vi "UHR-Fleezers Control (host) - 16.2.2v2.vi"() -> ()   [LabVIEW 2014]
uses:
  <vilib>/rvi/interface/nirviMethod/nirviMethod.xnode
  <vilib>/rvi/interface/nirviCloseFPGA/nirviCloseFPGA.xnode
  <vilib>/express/express analysis/Spectral/XNode/ExpressSpectralMeasurementsBlockNode.xnode
  <vilib>/rvi/interface/nirviReadWriteControl/nirviReadWriteControl.xnode
  <vilib>/Analysis/NI_AALBase.lvlib
  <vilib>/express/express analysis/Spectral/Block/exnSpectralBlock spectral measurements PSD poly.vi
  <vilib>/rvi/interface/nirviOpenFPGA/nirviOpenFPGA.xnode
  <vilib>/Platform/TimedLoop/XDataNode/XDataNode.xnode
  <vilib>/Platform/TimedLoop/XDataNode/nitl_modes.ctl
  <vilib>/Platform/TimedLoop/XDataNode/XDNodeRunTimeDep.lvlib
  <vilib>/Platform/TimedLoop/XDataNode/wakeup.ctl
  <vilib>/Platform/TimedLoop/XDataNode/timing_clust.ctl
  <vilib>/Utility/miscctls.llb/LVPoint32TypeDef.ctl
  <vilib>/userdefined/High Color/nirio_resource_hc.ctl
  openfpgaref.8.6.ctl
  <vilib>/Utility/miscctls.llb/LVMinMaxIncTypeDef.ctl
  <vilib>/vision/NI_Vision_Development_Module.lvlib
  <vilib>/Instr/_visa.llb/VISA Configure Serial Port (Instr).vi
  <vilib>/rvi/errors/niLvFpgaMergeErrorWithErrorCode.vi
  <vilib>/Analysis/baseanly.llb/Mean (DBL).vi
  Duncan Nall/Fluorescence simulation/Global for fluorescence simulation mean (30 samples), (power series).vi
  <vilib>/addons/database/NI_Database_API.lvlib
  <vilib>/vision/Avi.llb/IMAQ AVI2 Refnum.ctl
  <vilib>/gmath/NI_Gmath.lvlib
  <vilib>/addons/database/Connection.llb/DB Tools Open Connec (Path).vi
  <vilib>/sound2/lvsound2.llb/Sound Output Write (DBL Single).vi
  <vilib>/Waveform/WDTOps.llb/WDT Append Waveforms DBL.vi
  <vilib>/express/express analysis/Spectral/Block/exnSpectralBlock spectral measurements PSD WFM.vi
  <vilib>/Waveform/WDTOps.llb/WDT Index Channel DBL.vi
  <vilib>/rvi/errors/niLvFpgaAdjustHostInterfaceError.vi
  <vilib>/FPGAPlugInAG/PCIe-7852R/niLvFpga_ConfigureFifo_PCIe-7852R.vi
  <vilib>/FPGAPlugInAG/PCIe-7852R/niLvFpga_ReadFifo_PCIe-7852R.vi
  <vilib>/FPGAPlugInAG/PCIe-7852R/niLvFpga_Open_PCIe-7852R.vi
  openfpgaref.initrf.ctl
  FPGA Bitfiles/UHR-FleezersInst_FPGATarget_intitializeRFsyn_v1.lvbitx
  <vilib>/FPGAPlugInAG/PCIe-7852R/niLvFpga_Close_PCIe-7852R.vi
  FPGA Bitfiles/UHR-FleezersInst_FPGATarget_UHR-Fleezers_main_16.2.1v3.lvbitx
  <vilib>/FPGAPlugInAG/PCIe-7852R/niLvFpga_Reset_PCIe-7852R.vi
  <vilib>/FPGAPlugInAG/PCIe-7852R/niLvFpga_Run_PCIe-7852R.vi
  NiFpgaLv.dll
  <vilib>/Utility/error.llb/Error Cluster From Error Code.vi
  FPGA Bitfiles/UHR-FleezersInst_FPGATarget_UHR-FleezersCont_RmCmolmxQJQ.lvbitx
  UHR-Fleezers Control (fpga) - avogadro 3.vi
  <vilib>/FPGAPlugInAG/PCIe-7852R/niLvFpga_StopFifo_PCIe-7852R.vi
  <vilib>/FPGAPlugInAG/PCIe-7852R/niLvFpga_StartFifo_PCIe-7852R.vi
  <vilib>/addons/database/Connection.llb/Conn ObjectReference.ctl
  <vilib>/sound2/lvsound2.llb/Sampling Mode.ctl
  <vilib>/sound2/lvsound2.llb/Sound Data Format.ctl
panel:
  out "Read offset current":string(combo)
  out "PSD Y Sum":dbl[](array[numeric])
  out "log file ref":refnum<file>
  out "AL Running":bool
  in  "AL Delay (s)":u32
  in  "Stop assembly line":bool
  in  "Cy5 Fl.  Thresh. (kHz)":dbl=24.5
  in  "Cy3 Fl.  Thresh. (kHz)":dbl=19.0
  in  "Get Fluorophore":bool
  in  "X or Y?":bool=TRUE
  out "Red Fluorophore":bool
  out "Green Fluorophore":bool
  in  "Numeric":dbl
  in  "stop":bool
  in  "Start assembly line":bool
  out "Sigma/Mean 3":dbl=nan caption="Sigma/Mean" format="%#_2g"
  out "Rate sigma (Hz) 3":dbl caption="Sigma (Hz)" format="%0.2f"
  out "APD 3 Rate (Hz)":dbl format="%#_3p"
  out "HP3 Flush Time (s)":dbl=90.0
  out "HP1 Flush Time (s)":dbl=60.0
  out "TTrig":cluster{dbl, dbl}(graph)
  in  "Sample Channel\nFlow":bool
  in  "Inject Pump 1":bool
  in  "Inject Pump 3":bool
  in  "Pump 1 contents":string="Bottom: DNA beads" caption="Contents"
  in  "Pump 3 contents":string="Top: ADig beads" caption="Contents"
  out "Time (s)":dbl=276.59999999999997
  in  "Index":dbl=1.0 caption="Save File Index" min=1.0 step=1.0
  in  "Scripts":T1(tab)
  in  "Fixed Traps Data\nScript":bool
  in  "Dump spot flow on?":bool=TRUE caption="Flow ON?"
  in  "Daq spot flow on":bool=TRUE caption="Flow ON?"
  in  "Cap 1 Samp Flow ON":bool=TRUE
  in  "Cap 2 Samp Flow ON":bool=TRUE
  in  "Got DNA bead":bool
  in  "Got ADig bead":bool
  in  "Cap 2 Flow ON":bool=TRUE
  in  "Cap 1 Flow ON":bool=TRUE
  in  "Cap 2 T ON":bool=TRUE
  in  "Move Cap. 2 (ADig Top)":bool
  in  "Move Cap. 1 (DNA Bottom)":bool
  in  "Cal/Data Acq. Spot":bool
  in  "Dump Beads":bool
  in  "Cap 1 T ON":bool=TRUE
  in  "Force FB Data\nScript":bool
  in  "Cap. 2 BD T1?\n(ADig T1, DNA T2)":bool
  in  "Active cal after cal?":bool
  in  "Fish after cal?":bool=TRUE
  in  "Flow ON during cal?":bool
  in  "Offset 2 Set":dbl=2.0
  in  "Offset 1 Set":dbl
  in  "Cal @ (MHz)":dbl=17.0
  in  "W/ Offset 1":bool=TRUE
  in  "Offset 1 Start (MHz)":dbl=12.0
  in  "W/ Offset 2":bool
  in  "Offset 2 Start (MHz)":dbl=16.0
  in  "Cal Stage Position":i32=3
  in  "Only check fixed trap T2":bool
  in  "Flow ON after\ntether testing?":bool=TRUE
  in  "Flow ON during \nfishing?":bool=TRUE
  in  "Fish again after \nraster break?":bool
  in  "Furthest Delta (MHz)":dbl=15.25 step=0.25
  in  "Green ON During Raster":bool
  in  "Move to Delta 2 (MHz)":dbl=12.3
  in  "Attempt Limit":dbl=15.0 caption="Limit"
  out "Attempts":dbl=2.0
  in  "Wait Before Save (s)":u32=1
  in  "Closest Delta (MHz)":dbl=10.5 step=0.25
  in  "Stop F (pN)":dbl=3.0
  in  "Then...":string(combo)="5"
  in  "Move to Delta 1 (MHz)":dbl=12.3
  in  "Tether Alarm?":bool=TRUE
  out "Tether":bool
  in  "TA Cancel Save?":bool
  in  "TA Green Off?":bool
  in  "Raster Set Upon Tether":u32=5
  in  "Save at end (5, 6)":bool
  in  "Stop Fishing When Tether":bool=TRUE
  in  "Delay before dipping (s)":dbl=5.0
  in  "Start dipping after?":bool
  in  "Green ON after FB ON?":bool
  in  "Remove Action Offset":bool
  in  "Stage Position To Establish FB":i32=3
  in  "Trap Trig Fl.":bool
  in  "Starting \nTrap Delta (MHz)":dbl=15.25
  in  "Trap Delta Before Moving":dbl=13.0
  in  "Wait (s)":u32=1
  in  "Green ON":bool
  in  "Start dipping after?":bool=TRUE
  in  "Fixed Traps Trap Delta (MHz)":dbl=15.25 caption="Trap Delta (MHz)"
  out "TTrig Fin Thresh (nm)":dbl
  out "TTrig Sig (nm)":dbl
  out "Threshold stored (nm)":dbl
  in  "Neg. TTrig FPGA":bool=TRUE
  in  "Test ttrig":bool
  in  "Trap Trig. (FPGA)":bool=TRUE
  out "Initializing":bool
  in  "Reinitialize":bool
  out "Triggered":bool
  out "Waiting":bool
  in  "Trap Trig. Fl.":bool
  in  "Wait to get offset (n)":u32=10
  in  "Threshold (nm)":dbl=15.0
  in  "Fl. ON time (n)":i32=90
  out "T1 x pos data":dbl[](array[numeric])=[-9.744913000165011, -9.744913000165011]
  out "max value":dbl=-0.9003514563721442
  out "min value":dbl=-1.184251119672945
  in  "Mean T1 Position\nto compare (nm)":dbl caption="Mean T1 for Comparison (nm)" format="%0.2f"
  out "mean":dbl=-1.0423012880225446 format="%0.2f"
  out "standard\ndeviation":dbl=0.2007473770965739 format="%0.2f"
  out "TTrig Sig (Int)":i64
  out "TTrig Fin Thresh (Int)":i64
  in  "FB Trig Integrate":u32=1
  in  "Green ON\nafter start\nreturn?":bool
  in  "Green delay after \nstart return (s)":dbl
  out "Dwell Time (s)":dbl
  in  "FB OFF when \nflow ON":bool
  in  "Flow ON \nduring return\nfrom dip?":bool=TRUE
  in  "Flow ON\nduring daq?":bool=TRUE
  in  "Flow ON\nduring dip?":bool=TRUE
  in  "Cancel dwell":bool
  in  "Pause dwell":bool
  in  "Dwell Duration (s)":i32=45
  in  "Green ON\nbefore dip?":bool
  in  "Cont. Repeat Dipping?":bool=TRUE
  in  "Dipping Delta (MHz)":dbl=15.0
  in  "Move trap \nbefore dip move?":bool
  in  "Save data after return?":bool
  in  "Green ON \nafter return?":bool=TRUE
  in  "Dip Trap Delta 2 (MHz)":dbl=15.0
  in  "Move trap after return?":bool
  in  "Dip Duration (s)":i32=15
  in  "Dip for Protein":bool
  in  "Dip Stage \nPosition":i32=5
  in  "Return Stage \nPosition":i32=3
  out "Dip Time (s)":i32=16
  out "Dip #":i32=5
  in  "Y change (mm)":dbl=-3.0
  in  "Profile":bool
  out "Current Position":cluster{dbl, dbl, dbl}={1.6, 0.50781, -0.0311}
  in  "Shift confocal":bool
  in  "Auto F Reset":bool
  in  "Yank when?":bool
  in  "Yank to which?":bool
  in  "Yank to SP":dbl[](array[numeric])=[-0.128, -0.158, -0.183, -0.21, -0.01, -0.0319, -0.094, -0.143]
  in  "APD to Watch":bool
  out "Duration (s)":dbl=8.399999999999977
  in  "Action":string(combo)="Yank"
  in  "Fl. Triggered...":bool
  in  "Fl. Delta Thresh. (kHz)":dbl=0.14
  out "Waiting":bool
  out "Fl. High":bool
  in  "N pts to average":u16=6
  in  "Yank Delay (s)":dbl=3.0
  in  "Yank to Trap Delta (MHz)":dbl[](array[numeric])=[16.3, 15.85, 14.85]
  in  "N Array El":u8=4 min=1 step=1
  in  "Random Choice":bool=TRUE
  in  "Force Yank":bool
  in  "Reset Force":bool
  in  "N Steps":dbl=20.0
  in  "Step Size (nm)":dbl=0.34
  in  "Save ave factor":dbl=1.0
  in  "Take Stepping Data":bool
  in  "Cancel slow trap scan":bool
  out "Scanning (slow scan)":bool caption="Scanning"
  in  "Start slow trap scan":bool
  in  "Trap step dwell (ms) (slow scan)":dbl=20.0 caption="Trap step dwell (ms)"
  in  "Trap step increment (MHz) (slow scan)":dbl=0.01 caption="Trap step increment (MHz)"
  in  "Trap scan range (MHz) (slow scan)":dbl=2.5 caption="Trap scan range (MHz)"
  in  "Duration 2 (s)":dbl=60.0
  in  "Stop saving when done":bool=TRUE
  in  "Trap pause durations (s)":dbl[](array[numeric])=[20.0, 20.0, 20.0] format="%.1f"
  in  "No pause on first pull":bool=TRUE
  in  "Start slow f-ext":bool
  in  "Pause scan":bool
  in  "Stop pulling and reverse":bool
  in  "Stop at pause on pull":bool=TRUE
  in  "Cancel pause":bool
  in  "Immediately quit scan":bool
  out "Scanning (slow scan) 2":bool caption="Scanning"
  in  "Trap step increment (MHz) (slow scan) 2":dbl=0.01 caption="Trap step increment (MHz)"
  in  "Trap step dwell (ms) (slow scan) 2":dbl=200.0 caption="Trap step dwell (ms)"
  in  "Pause after pull, before next relax":bool=TRUE
  in  "Stop at pause on relax":bool=TRUE
  in  "Pause after relax, before next pull":bool=TRUE
  in  "Finish scan and quit":bool
  in  "Repeat n pull/relax scans":dbl=10.0
  in  "Trap pause positions (MHz)":dbl[](array[numeric])=[12.6, 13.69, 15.09] min=0.0 max=20.0 step=1e-05 format="%.4g"
  in  "Read trap position file first":bool
  out "Read trap position error":errorcluster
  in  "Start saving before pull":bool
  out "Sigma/Mean 2":dbl=nan caption="Sigma/Mean" format="%#_2g"
  out "Rate sigma (Hz) 2":dbl caption="Sigma (Hz)" format="%0.2f"
  out "APD 2 Rate (Hz)":dbl format="%#_3p"
  out "Primary Video Display":T2(plugin-control)
  out "Waveform Graph":dbl[](graph) caption="APD Line Scan"
  out "Messages":string="5:45 PM\tUHR-Fleezers ready.\r"
  in  "APD Ave N":dbl=20.0 caption="DMA sets to ave"
  out "Int. Time (s)":dbl=6.0
  in  "Stop All":bool=TRUE
  out "Sigma/Mean":dbl=nan format="%#_2g"
  out "Rate sigma (Hz)":dbl caption="Sigma (Hz)" format="%0.2f"
  in  "Tab Control 6":T3(tab)
  in  "APD 3 Offset":dbl
  in  "APD 2 Offset":dbl
  in  "APD 1 Offset":dbl
  out "RMS (Ang)":dbl=nan format="%_2g"
  in  "Bead Sep. Int. Time (s)":dbl=3.0 caption="Int. Time (s)"
  in  "Below (kHz)":dbl=1.0
  in  "Above (kHz)":dbl=2.0
  in  "Adjust Scale\nto Mean":bool
  in  "Remove Offset":bool
  in  "Offset (nm)":dbl=-102.44041120379248 format="%#_3g"
  out "Mean":dbl=nan caption="Mean (pN)" format="%#_3g"
  out "Force":waveform(dbl)[](graph)=[{"t0"=timestamp(13.800000000000011 s since 1904-01-01), "dt"=0.15, "Y"=[-inf, -inf], "attributes"=variant("NI_ChannelName"=variant(string "T1 X"))}, {"t0"=timestamp(13.800000000000011 s since 1904-01-01), "dt"=0.15, "Y"=[inf, inf], "attributes"=variant("NI_ChannelName"=variant(string "T2 X"))}]
  out "APD Chart":waveform(dbl)[](graph)=[{"t0"=timestamp(13.800000000000011 s since 1904-01-01), "dt"=0.15, "Y"=[0.0, 0.0], "attributes"=variant("NI_ChannelName"=variant(string "APD 1"))}, {"t0"=timestamp(13.800000000000011 s since 1904-01-01), "dt"=0.15, "Y"=[0.0, 0.0], "attributes"=variant("NI_ChannelName"=variant(string "APD 2"))}]
  in  "Calibration":u16(ring)=2 items=["None", "Position", "Force"]
  out "T1 X":dbl=-inf caption="T1 X (pN)" format="%0.2f"
  out "T2 X":dbl=-inf caption="T2 X (pN)" format="%0.2f"
  out "Bead Separation":waveform(dbl)(graph)={"t0"=timestamp(13.800000000000011 s since 1904-01-01), "dt"=0.15, "Y"=[nan, nan], "attributes"=variant("NI_ChannelName"=variant(string "T1 X"))}
  out "Bead Mean (nm)":dbl=nan caption="Mean (nm)" format="%0.2f"
  out "Difference":dbl=-inf caption="Difference (pN)" format="%.2g"
  out "Confocal Y 2 (V)":dbl=6.809280068361465
  out "Confocal X 2 (V)":dbl=0.7223435163426621
  out "Confocal Y 1 (V)":dbl=7.15854518265328
  out "Confocal X 1 (V)":dbl=0.3727259132663963
  in  "Set High F Confocal Spot (X-Y)":bool
  in  "Take Detection Laser\nImage":bool
  out "APD 2":T2(plugin-control) caption="APD 2 (Cy5)"
  in  "Flip Green Filter":bool
  in  "Set X Only":bool
  in  "Set Y Only":bool
  out "APD 1":T2(plugin-control) caption="APD 1 (Cy3)"
  out "Detection Laser Y":T2(plugin-control)
  out "Pointer Y (V)":dbl=7.15854518265328 format="%_3g"
  out "Pointer X (V)":dbl=0.3727259132663963 format="%_3g"
  in  "Set Confocal Spot (X-Y)":bool
  out "Detection Laser X":T2(plugin-control)
  out "APD 3":T2(plugin-control) caption="APD 3 (Cy2)"
  in  "Display Saved Data":string(combo)
  out "Saved trap pos":dbl[](graph)
  out "Saved APD":dbl[][](graph)=[[340.0, 553.3333333333334, 453.33333333333337, 406.6666666666667, 466.6666666666667, 473.33333333333337, 466.6666666666667, 640.0, 586.6666666666667, 573.3333333333334, 540.0, 473.33333333333337, 473.33333333333337, 480.0, 413.33333333333337, 566.6666666666667, 560.0, 480.0, 540.0, 526.6666666666667, 553.3333333333334, 526.6666666666667, 526.6666666666667, 560.0, 360.0, 420.0, 533.3333333333334, 620.0, 580.0, 500.0, 620.0, 466.6666666666667, 646.6666666666667, 626.6666666666667, 466.6666666666667, 520.0, 506.6666666666667, 553.3333333333334, 593.3333333333334, 546.6666666666667, 446.6666666666667, 573.3333333333334, 506.6666666666667, 526.6666666666667, 546.6666666666667, 626.6666666666667, 573.3333333333334, 540.0, 466.6666666666667, 506.6666666666667, 520.0, 646.6666666666667, 620.0, 533.3333333333334, 460.0, 513.3333333333334, 460.0, 386.6666666666667, 553.3333333333334, 440.0, 466.6666666666667, 506.6666666666667, 500.0, 546.6666666666667, 533.3333333333334, 473.33333333333337, 440.0, 560.0, 513.3333333333334, 600.0, 480.0, 386.6666666666667, 606.6666666666667, 413.33333333333337, 500.0, 426.6666666666667, 520.0, 620.0, 540.0, 566.6666666666667, 613.3333333333334, 580.0, 766.6666666666667, 786.6666666666667, 860.0, 1126.6666666666667, 1426.6666666666667, 1733.3333333333335, 1826.6666666666667, 2453.3333333333335, 2100.0, 2406.666666666667, 2826.666666666667, 4160.0, 2906.666666666667, 2893.3333333333335, 3046.666666666667, 3060.0, 3160.0, 2666.666666666667, 3166.666666666667, 3353.3333333333335, 3086.666666666667, 3613.3333333333335, 3966.666666666667, 3993.3333333333335, 3546.666666666667, 3326.666666666667, 3440.0, 3126.666666666667, 3580.0, 3073.3333333333335, 3306.666666666667, 3220.0, 2666.666666666667, 2926.666666666667, 2993.3333333333335, 3046.666666666667, 3086.666666666667, 3513.3333333333335, 2940.0, 3140.0, 3406.666666666667, 3380.0, 3153.3333333333335, 3053.3333333333335, 3453.3333333333335, 3626.666666666667, 2666.666666666667, 2566.666666666667, 2513.3333333333335, 2560.0, 2493.3333333333335, 2760.0, 2220.0, 2606.666666666667, 3100.0, 2333.3333333333335, 2613.3333333333335, 2673.3333333333335, 2480.0, 2546.666666666667, 2633.3333333333335, 2746.666666666667, 2786.666666666667, 2806.666666666667, 2340.0, 2613.3333333333335, 2273.3333333333335, 2660.0, 2853.3333333333335, 3160.0, 3280.0, 2633.3333333333335, 2360.0, 3113.3333333333335, 3233.3333333333335, 2793.3333333333335, 2980.0, 3080.0, 2500.0, 3026.666666666667, 3233.3333333333335, 2820.0, 2900.0, 2506.666666666667, 3146.666666666667, 2806.666666666667, 2560.0, 2560.0, 2620.0, 2780.0, 3266.666666666667, 3260.0, 2593.3333333333335, 2773.3333333333335, 2440.0, 3106.666666666667, 2640.0, 2900.0, 2793.3333333333335, 2906.666666666667, 3326.666666666667, 2926.666666666667, 3060.0, 3560.0, 3046.666666666667, 2746.666666666667, 2560.0, 2740.0, 3600.0, 4053.3333333333335, 2666.666666666667, 2940.0, 2166.666666666667, 2626.666666666667, 2593.3333333333335, 5833.333333333334, 3986.666666666667, 3573.3333333333335, 3973.3333333333335, 4106.666666666667, 3453.3333333333335, 3046.666666666667, 3240.0, 2973.3333333333335, 3420.0, 3080.0, 2753.3333333333335, 2973.3333333333335, 2940.0, 3040.0, 3680.0, 3653.3333333333335, 3533.3333333333335, 3486.666666666667, 3693.3333333333335, 3393.3333333333335, 2746.666666666667, 3360.0, 2753.3333333333335, 3313.3333333333335, 3246.666666666667, 3800.0, 3286.666666666667, 3513.3333333333335, 2493.3333333333335, 2546.666666666667, 2860.0, 2426.666666666667, 2733.3333333333335, 2426.666666666667, 2353.3333333333335, 2993.3333333333335, 2186.666666666667, 2420.0, 2460.0, 2366.666666666667, 2613.3333333333335, 3453.3333333333335, 2653.3333333333335, 2640.0, 2853.3333333333335, 2873.3333333333335, 2546.666666666667, 2526.666666666667, 2426.666666666667, 2573.3333333333335, 2700.0, 2046.6666666666667, 2926.666666666667, 2506.666666666667, 2253.3333333333335, 2733.3333333333335, 2633.3333333333335, 3240.0, 2620.0, 2740.0, 2686.666666666667, 2660.0, 3460.0, 2793.3333333333335, 4280.0, 2606.666666666667, 3593.3333333333335, 3386.666666666667, 2893.3333333333335, 3073.3333333333335, 2713.3333333333335, 2680.0, 5340.0, 2920.0, 2660.0, 2913.3333333333335, 2613.3333333333335, 2793.3333333333335, 3073.3333333333335, 2580.0, 2733.3333333333335, 3086.666666666667, 2546.666666666667, 2720.0, 2840.0, 3193.3333333333335, 2413.3333333333335, 2653.3333333333335, 2566.666666666667, 3240.0, 3226.666666666667, 2486.666666666667, 2393.3333333333335, 2680.0, 2726.666666666667, 2406.666666666667, 3093.3333333333335, 2573.3333333333335, 3033.3333333333335, 2633.3333333333335, 3200.0, 2853.3333333333335, 2913.3333333333335, 3080.0, 2340.0, 2386.666666666667, 2626.666666666667, 2680.0, 2700.0, 2440.0, 2693.3333333333335, 2880.0, 2753.3333333333335, 2753.3333333333335, 2493.3333333333335, 4826.666666666667, 2013.3333333333335, 2366.666666666667, 2573.3333333333335, 3046.666666666667, 2693.3333333333335, 2373.3333333333335, 2700.0, 2580.0, 2140.0, 2573.3333333333335, 2520.0, 2406.666666666667, 2766.666666666667, 2366.666666666667, 2393.3333333333335, 2573.3333333333335, 2580.0, 2700.0, 2733.3333333333335, 2500.0, 2413.3333333333335, 2453.3333333333335, 2580.0, 2586.666666666667, 2066.666666666667, 2526.666666666667, 2066.666666666667, 2780.0, 2360.0, 2806.666666666667, 2686.666666666667, 2826.666666666667, 2473.3333333333335, 2660.0, 2693.3333333333335, 3293.3333333333335, 2653.3333333333335, 2893.3333333333335, 2766.666666666667, 2560.0, 2673.3333333333335, 2226.666666666667, 2240.0, 2300.0, 2473.3333333333335, 2680.0, 2573.3333333333335, 2353.3333333333335, 2906.666666666667, 2206.666666666667, 3213.3333333333335, 2580.0, 2500.0, 3126.666666666667, 3013.3333333333335, 2920.0, 3173.3333333333335, 2866.666666666667, 3100.0, 2720.0, 3260.0, 2666.666666666667, 3060.0, 2633.3333333333335, 2880.0, 3646.666666666667, 3740.0, 2966.666666666667, 2826.666666666667, 3046.666666666667, 3013.3333333333335, 2546.666666666667, 2733.3333333333335, 2373.3333333333335, 2920.0, 3240.0, 2433.3333333333335, 2653.3333333333335, 2400.0, 2146.666666666667, 2333.3333333333335, 2486.666666666667, 2760.0, 2573.3333333333335, 2180.0, 2506.666666666667, 2500.0, 2686.666666666667, 2180.0, 1966.6666666666667, 2673.3333333333335, 3273.3333333333335, 2840.0, 2606.666666666667, 2680.0, 2573.3333333333335, 2686.666666666667, 2913.3333333333335, 2853.3333333333335, 2706.666666666667, 2913.3333333333335, 3053.3333333333335, 3020.0, 2886.666666666667, 3006.666666666667, 2446.666666666667, 2966.666666666667, 2866.666666666667, 2740.0, 3746.666666666667, 3073.3333333333335, 3460.0, 2453.3333333333335, 2520.0, 2406.666666666667, 2786.666666666667, 2626.666666666667, 2520.0, 2593.3333333333335, 2780.0, 2786.666666666667, 2340.0, 2600.0, 2266.666666666667, 2780.0, 2600.0, 2586.666666666667, 2773.3333333333335, 2560.0, 2566.666666666667, 1946.6666666666667, 2393.3333333333335, 2733.3333333333335, 4080.0, 2320.0, 2453.3333333333335, 2380.0, 2446.666666666667, 2773.3333333333335, 2500.0, 2433.3333333333335, 2793.3333333333335, 2880.0, 2373.3333333333335, 3006.666666666667, 2540.0, 2353.3333333333335, 3626.666666666667, 2393.3333333333335, 2773.3333333333335, 2900.0, 2993.3333333333335, 2460.0, 2533.3333333333335, 2426.666666666667, 2286.666666666667, 2293.3333333333335, 2380.0, 3153.3333333333335, 2473.3333333333335, 2520.0, 2940.0, 2626.666666666667, 2640.0, 2793.3333333333335, 2646.666666666667, 2446.666666666667, 2913.3333333333335, 3066.666666666667, 2666.666666666667, 2853.3333333333335, 3026.666666666667, 2306.666666666667, 2860.0, 2473.3333333333335, 2733.3333333333335, 2333.3333333333335, 4120.0, 2433.3333333333335, 1926.6666666666667, 2386.666666666667, 2740.0, 2713.3333333333335, 2500.0, 2686.666666666667, 2533.3333333333335, 2073.3333333333335, 2286.666666666667, 2420.0, 2933.3333333333335, 2640.0, 2953.3333333333335, 2933.3333333333335, 2826.666666666667, 3033.3333333333335, 2566.666666666667, 2906.666666666667, 3013.3333333333335, 2586.666666666667, 2360.0, 2360.0, 2380.0, 2566.666666666667, 3153.3333333333335, 2360.0, 2433.3333333333335, 2520.0, 2826.666666666667, 2353.3333333333335, 2233.3333333333335, 2406.666666666667, 2920.0, 3513.3333333333335, 2920.0, 2840.0, 2606.666666666667, 2786.666666666667, 2606.666666666667, 2200.0, 2960.0, 2846.666666666667, 2640.0, 2526.666666666667, 2746.666666666667, 2660.0, 2246.666666666667, 2486.666666666667, 2566.666666666667, 2413.3333333333335, 2533.3333333333335, 2633.3333333333335, 2313.3333333333335, 2373.3333333333335, 2646.666666666667, 2826.666666666667, 2446.666666666667, 2620.0, 3006.666666666667, 2353.3333333333335, 2433.3333333333335, 2580.0, 2413.3333333333335, 3160.0, 2166.666666666667, 2226.666666666667, 2586.666666666667, 2266.666666666667, 2306.666666666667, 2700.0, 3140.0, 3966.666666666667, 3353.3333333333335, 3426.666666666667, 3393.3333333333335, 3680.0, 3066.666666666667, 3400.0, 3000.0, 2946.666666666667, 2553.3333333333335, 2573.3333333333335, 2446.666666666667, 2513.3333333333335, 2100.0, 2153.3333333333335, 3406.666666666667, 2733.3333333333335, 3220.0, 2960.0, 3240.0, 2666.666666666667, 3026.666666666667, 2893.3333333333335, 2646.666666666667, 3120.0, 3033.3333333333335, 3233.3333333333335, 2300.0, 2646.666666666667, 3133.3333333333335, 2660.0, 3693.3333333333335, 2686.666666666667, 3420.0, 3373.3333333333335, 3240.0, 2973.3333333333335, 2726.666666666667, 3273.3333333333335, 3720.0, 2960.0, 3240.0, 3020.0, 3226.666666666667, 2953.3333333333335, 3286.666666666667, 2946.666666666667, 5333.333333333334, 3393.3333333333335, 3053.3333333333335, 3413.3333333333335, 3386.666666666667, 3366.666666666667, 3800.0, 3173.3333333333335, 3266.666666666667, 3480.0, 3206.666666666667, 3473.3333333333335, 4853.333333333334, 3740.0, 3266.666666666667, 4133.333333333334, 3046.666666666667, 3673.3333333333335, 3006.666666666667, 3026.666666666667, 4026.666666666667, 2973.3333333333335, 3233.3333333333335, 3333.3333333333335, 3200.0, 2500.0, 2893.3333333333335, 3006.666666666667, 2946.666666666667, 2540.0, 2633.3333333333335, 2686.666666666667, 2846.666666666667, 3126.666666666667, 3053.3333333333335, 2973.3333333333335, 3240.0, 2906.666666666667, 3266.666666666667, 2733.3333333333335, 2646.666666666667, 2886.666666666667, 3200.0, 2486.666666666667, 2966.666666666667, 2466.666666666667, 2686.666666666667, 2806.666666666667, 3673.3333333333335, 3080.0, 2753.3333333333335, 2773.3333333333335, 2893.3333333333335, 2940.0, 2933.3333333333335, 3253.3333333333335, 3060.0, 3446.666666666667, 3060.0, 3393.3333333333335, 2953.3333333333335, 3333.3333333333335, 2760.0, 2580.0, 3673.3333333333335, 3100.0, 2880.0, 3073.3333333333335, 3013.3333333333335, 2973.3333333333335, 2946.666666666667, 3160.0, 3526.666666666667, 2726.666666666667, 2986.666666666667, 2926.666666666667, 2840.0, 2986.666666666667, 3353.3333333333335, 2906.666666666667, 3906.666666666667, 4086.666666666667, 2626.666666666667, 2606.666666666667, 3360.0, 2780.0, 3220.0, 3653.3333333333335, 3973.3333333333335, 3853.3333333333335, 3033.3333333333335, 3593.3333333333335, 3420.0, 4353.333333333334, 3553.3333333333335, 3593.3333333333335, 3713.3333333333335, 3733.3333333333335, 4480.0, 2713.3333333333335, 2500.0, 2946.666666666667, 2886.666666666667, 3246.666666666667, 3206.666666666667, 3326.666666666667, 2873.3333333333335, 2680.0, 2953.3333333333335, 3226.666666666667, 3373.3333333333335, 2933.3333333333335, 2973.3333333333335, 2980.0, 2973.3333333333335, 7133.333333333334, 3386.666666666667, 3306.666666666667, 3600.0, 2273.3333333333335, 2466.666666666667, 2573.3333333333335, 2706.666666666667, 2286.666666666667, 3073.3333333333335, 2753.3333333333335, 2746.666666666667, 2500.0, 2660.0, 2093.3333333333335, 2546.666666666667, 2866.666666666667, 1946.6666666666667, 2600.0, 2380.0, 2320.0, 1926.6666666666667, 2146.666666666667, 2513.3333333333335, 2666.666666666667, 2366.666666666667, 2560.0, 2313.3333333333335, 2480.0, 2620.0, 2706.666666666667, 2760.0, 2773.3333333333335, 2853.3333333333335, 2313.3333333333335, 2726.666666666667, 2506.666666666667, 2546.666666666667, 2566.666666666667, 2533.3333333333335, 3046.666666666667, 2240.0, 2680.0, 2706.666666666667, 2360.0, 2500.0, 2300.0, 2520.0, 2366.666666666667, 2446.666666666667, 2860.0, 2393.3333333333335, 2626.666666666667, 2046.6666666666667, 2573.3333333333335, 2666.666666666667, 3066.666666666667, 2486.666666666667, 2453.3333333333335, 3226.666666666667, 2840.0, 2600.0, 2526.666666666667, 2693.3333333333335, 2566.666666666667, 2800.0, 2533.3333333333335, 2620.0, 2946.666666666667, 2280.0, 2600.0, 3806.666666666667, 3566.666666666667, 3460.0, 2673.3333333333335, 2506.666666666667, 2273.3333333333335, 2393.3333333333335, 2233.3333333333335, 2006.6666666666667, 2586.666666666667, 2300.0, 2233.3333333333335, 2386.666666666667, 1913.3333333333335, 2466.666666666667, 2326.666666666667, 2153.3333333333335, 2420.0, 2680.0, 2666.666666666667, 2613.3333333333335, 2806.666666666667, 3033.3333333333335, 2286.666666666667, 2453.3333333333335, 2540.0, 2540.0, 2480.0, 2646.666666666667, 2526.666666666667, 2433.3333333333335, 2620.0, 3180.0, 2520.0, 2900.0, 2860.0, 3446.666666666667, 3246.666666666667, 3233.3333333333335, 3346.666666666667, 2866.666666666667, 2720.0, 3040.0, 2580.0, 3213.3333333333335, 3780.0, 2900.0, 2533.3333333333335, 2873.3333333333335, 2480.0, 2066.666666666667, 3020.0, 2820.0, 2720.0, 2213.3333333333335, 2300.0, 2486.666666666667, 2680.0, 2673.3333333333335, 2993.3333333333335, 2673.3333333333335, 2513.3333333333335, 2920.0, 2886.666666666667, 2620.0, 2773.3333333333335, 2873.3333333333335, 2393.3333333333335, 2313.3333333333335, 2326.666666666667, 2293.3333333333335, 2073.3333333333335, 2760.0, 2120.0, 2493.3333333333335, 2993.3333333333335, 2886.666666666667, 2693.3333333333335, 2226.666666666667, 2420.0, 2493.3333333333335, 2873.3333333333335, 2740.0, 2900.0, 3306.666666666667, 2560.0, 2833.3333333333335, 2486.666666666667, 2300.0, 3020.0, 2453.3333333333335, 2566.666666666667, 2626.666666666667, 2460.0, 2560.0, 2486.666666666667, 2266.666666666667, 2366.666666666667, 3026.666666666667, 2653.3333333333335, 2800.0, 2666.666666666667, 2360.0, 2640.0, 2740.0, 2806.666666666667, 3253.3333333333335, 3580.0, 3760.0, 3560.0, 3533.3333333333335, 2946.666666666667, 3213.3333333333335, 3166.666666666667, 3020.0, 3280.0, 3840.0, 2873.3333333333335, 2913.3333333333335, 3093.3333333333335, 2846.666666666667, 2893.3333333333335, 3500.0, 3246.666666666667, 3313.3333333333335, 3020.0, 2926.666666666667, 2246.666666666667, 1933.3333333333335, 2653.3333333333335, 2173.3333333333335, 2460.0, 2606.666666666667, 2653.3333333333335, 2633.3333333333335, 2540.0, 2513.3333333333335, 2653.3333333333335, 2446.666666666667, 2646.666666666667, 2680.0, 2666.666666666667, 2766.666666666667, 3066.666666666667, 2833.3333333333335, 2933.3333333333335, 2446.666666666667, 2513.3333333333335, 2746.666666666667, 2833.3333333333335, 2666.666666666667, 2533.3333333333335, 2806.666666666667, 2526.666666666667, 2326.666666666667, 2586.666666666667, 2300.0, 2720.0, 2413.3333333333335, 2393.3333333333335, 2400.0, 2640.0, 2393.3333333333335, 2173.3333333333335, 2033.3333333333335, 2073.3333333333335, 1953.3333333333335, 2280.0, 2033.3333333333335, 2293.3333333333335, 2193.3333333333335, 2533.3333333333335, 2566.666666666667, 2306.666666666667, 2400.0, 2366.666666666667, 1980.0, 2126.666666666667, 2166.666666666667, 2606.666666666667, 2426.666666666667, 2566.666666666667, 2533.3333333333335, 2740.0, 2653.3333333333335, 2286.666666666667, 2906.666666666667, 2406.666666666667, 2466.666666666667, 2026.6666666666667, 2373.3333333333335, 3306.666666666667, 2086.666666666667, 2320.0, 2520.0, 2100.0, 2320.0, 2506.666666666667, 2173.3333333333335, 2600.0, 2560.0, 2326.666666666667, 2173.3333333333335, 2853.3333333333335, 2760.0, 2646.666666666667, 2260.0, 2546.666666666667, 2660.0, 2300.0, 2340.0, 3200.0, 2520.0, 2613.3333333333335, 2513.3333333333335, 2113.3333333333335, 2540.0, 2753.3333333333335, 2293.3333333333335, 2453.3333333333335, 2580.0, 2793.3333333333335, 2446.666666666667, 2686.666666666667, 2820.0, 2360.0, 2100.0, 2240.0, 2440.0, 2553.3333333333335, 2353.3333333333335, 1860.0, 2040.0, 2340.0, 2320.0, 2706.666666666667, 2793.3333333333335, 2453.3333333333335, 2126.666666666667, 2206.666666666667, 2246.666666666667, 2660.0, 1993.3333333333335, 2520.0, 2040.0, 2626.666666666667, 2226.666666666667, 2406.666666666667, 2300.0, 2446.666666666667, 7433.333333333334, 2186.666666666667, 2760.0, 2620.0, 2486.666666666667, 2593.3333333333335, 2373.3333333333335, 2326.666666666667, 2333.3333333333335, 3006.666666666667, 3133.3333333333335, 4793.333333333334, 4653.333333333334, 2146.666666666667, 2900.0, 2400.0, 2286.666666666667, 2466.666666666667, 2520.0, 2673.3333333333335, 2593.3333333333335, 2453.3333333333335, 2660.0, 2793.3333333333335, 3293.3333333333335, 2240.0, 2313.3333333333335, 2446.666666666667, 2773.3333333333335, 2360.0, 3253.3333333333335, 2453.3333333333335, 2326.666666666667, 2293.3333333333335, 2460.0, 2586.666666666667, 2520.0, 2146.666666666667, 2080.0, 2606.666666666667, 2713.3333333333335, 2746.666666666667, 2353.3333333333335, 2266.666666666667, 2413.3333333333335, 2193.3333333333335, 2260.0, 2053.3333333333335, 2313.3333333333335, 2586.666666666667, 3573.3333333333335, 2646.666666666667, 2733.3333333333335, 2026.6666666666667, 2473.3333333333335, 2273.3333333333335, 2573.3333333333335, 2600.0, 2466.666666666667, 2753.3333333333335, 2360.0, 2433.3333333333335, 2126.666666666667, 2280.0, 2686.666666666667, 2386.666666666667, 2386.666666666667, 2720.0, 2153.3333333333335, 2613.3333333333335, 2206.666666666667, 2773.3333333333335, 2606.666666666667, 2626.666666666667, 2313.3333333333335, 2680.0, 2840.0, 2753.3333333333335, 2260.0, 2106.666666666667, 2480.0, 2473.3333333333335, 2313.3333333333335, 2986.666666666667, 2613.3333333333335, 2306.666666666667, 2573.3333333333335, 2220.0, 2546.666666666667, 2360.0, 2593.3333333333335, 2186.666666666667, 2493.3333333333335, 2346.666666666667, 2480.0, 2180.0, 2806.666666666667, 2600.0, 2460.0, 2493.3333333333335, 2093.3333333333335, 2840.0, 1993.3333333333335, 2820.0, 2333.3333333333335, 2213.3333333333335, 2300.0, 2426.666666666667, 2740.0, 2246.666666666667, 2853.3333333333335, 2726.666666666667, 3073.3333333333335, 2500.0, 2286.666666666667, 2413.3333333333335, 2853.3333333333335, 2573.3333333333335, 2553.3333333333335, 3100.0, 2880.0, 2753.3333333333335, 2793.3333333333335, 2666.666666666667, 2793.3333333333335, 2546.666666666667, 2400.0, 2573.3333333333335, 2506.666666666667, 2780.0, 2446.666666666667, 3026.666666666667, 2746.666666666667, 2606.666666666667, 2740.0, 2253.3333333333335, 2813.3333333333335, 2586.666666666667, 2760.0, 2286.666666666667, 2353.3333333333335, 2640.0, 2420.0, 2906.666666666667, 2593.3333333333335, 2626.666666666667, 2360.0, 2760.0, 2280.0, 2700.0, 2600.0, 2213.3333333333335, 2286.666666666667, 2133.3333333333335, 3066.666666666667, 2673.3333333333335, 1960.0, 2440.0, 2446.666666666667, 2506.666666666667, 2493.3333333333335, 2366.666666666667, 2613.3333333333335, 2546.666666666667, 2606.666666666667, 2553.3333333333335, 2213.3333333333335, 2346.666666666667, 2420.0, 2486.666666666667, 2646.666666666667, 2466.666666666667, 2553.3333333333335, 2186.666666666667, 2726.666666666667, 2193.3333333333335, 2800.0, 2360.0, 2980.0, 2300.0, 2593.3333333333335, 2706.666666666667, 2253.3333333333335, 2686.666666666667, 2660.0, 2426.666666666667, 2793.3333333333335, 2533.3333333333335, 2500.0, 2546.666666666667, 2380.0, 2473.3333333333335, 2400.0, 2606.666666666667, 2913.3333333333335, 2820.0, 2953.3333333333335, 2740.0, 2866.666666666667, 3086.666666666667, 3153.3333333333335, 2520.0, 2753.3333333333335, 2453.3333333333335, 3133.3333333333335, 2980.0, 2773.3333333333335, 2520.0, 2813.3333333333335, 2666.666666666667, 2626.666666666667, 2666.666666666667, 2826.666666666667, 2573.3333333333335, 3046.666666666667, 4160.0, 2526.666666666667, 2686.666666666667, 2753.3333333333335, 2533.3333333333335, 2680.0, 2633.3333333333335, 2206.666666666667, 2280.0, 2620.0, 2720.0, 3013.3333333333335, 3000.0, 2600.0, 2833.3333333333335, 3053.3333333333335, 2593.3333333333335, 2700.0, 3500.0, 2866.666666666667, 3000.0, 2546.666666666667, 2580.0, 2646.666666666667, 3553.3333333333335, 3213.3333333333335, 3106.666666666667, 2666.666666666667, 2926.666666666667, 2753.3333333333335, 3540.0, 2726.666666666667, 2906.666666666667, 2640.0, 2653.3333333333335, 2766.666666666667, 2426.666666666667, 2546.666666666667, 2720.0, 2426.666666666667, 2766.666666666667, 4460.0, 2413.3333333333335, 2586.666666666667, 2580.0, 2740.0, 2926.666666666667, 2906.666666666667, 2773.3333333333335, 2746.666666666667, 2553.3333333333335, 2813.3333333333335, 2893.3333333333335, 2793.3333333333335, 2693.3333333333335, 2926.666666666667, 3033.3333333333335, 2680.0, 2520.0, 2580.0, 2726.666666666667, 2186.666666666667, 2440.0, 2600.0, 2546.666666666667, 2553.3333333333335, 2040.0, 2166.666666666667, 2133.3333333333335, 2573.3333333333335, 2740.0, 2440.0, 2513.3333333333335, 2433.3333333333335, 2920.0, 2840.0, 3020.0, 2300.0, 2646.666666666667, 2480.0, 2540.0, 2780.0, 2940.0, 2526.666666666667, 2586.666666666667, 2320.0, 2040.0, 2853.3333333333335, 2680.0, 2960.0, 2426.666666666667, 2273.3333333333335, 5406.666666666667, 5646.666666666667, 2333.3333333333335, 2893.3333333333335, 2426.666666666667, 2593.3333333333335, 2780.0, 2433.3333333333335, 2593.3333333333335, 2360.0, 2240.0, 2280.0, 2240.0, 2273.3333333333335, 2040.0, 2206.666666666667, 2446.666666666667, 2293.3333333333335, 2453.3333333333335, 2093.3333333333335, 2200.0, 2346.666666666667, 2366.666666666667, 2600.0, 2340.0, 2280.0, 2046.6666666666667, 2480.0, 2660.0, 2620.0, 2033.3333333333335, 2800.0, 2346.666666666667, 2966.666666666667, 2393.3333333333335, 2726.666666666667, 2520.0, 2673.3333333333335, 2446.666666666667, 2553.3333333333335, 3006.666666666667, 2593.3333333333335, 2440.0, 2293.3333333333335, 2106.666666666667, 3006.666666666667, 2540.0, 2453.3333333333335, 1866.6666666666667, 2106.666666666667, 2106.666666666667, 2286.666666666667, 2246.666666666667, 2593.3333333333335, 2500.0, 2300.0, 2686.666666666667, 2753.3333333333335, 2853.3333333333335, 2393.3333333333335, 2686.666666666667, 2320.0, 3386.666666666667, 2626.666666666667, 2160.0, 2546.666666666667, 2333.3333333333335, 2826.666666666667, 2120.0, 2280.0, 3220.0, 1826.6666666666667, 2560.0, 2686.666666666667, 2560.0, 2680.0, 2200.0, 2193.3333333333335, 2100.0, 2520.0, 2480.0, 2546.666666666667, 2200.0, 2426.666666666667, 2513.3333333333335, 2206.666666666667, 2800.0, 2240.0, 2813.3333333333335, 2633.3333333333335, 2606.666666666667, 2400.0, 2380.0, 2793.3333333333335, 2306.666666666667, 2186.666666666667, 2500.0, 2560.0, 2166.666666666667, 1986.6666666666667, 2440.0, 2666.666666666667, 2706.666666666667, 2740.0, 2573.3333333333335, 2386.666666666667, 2793.3333333333335, 2333.3333333333335, 2206.666666666667, 2293.3333333333335, 2246.666666666667, 2680.0, 2486.666666666667, 2753.3333333333335, 2266.666666666667, 2953.3333333333335, 2040.0, 2313.3333333333335, 2646.666666666667, 3340.0, 2880.0, 2473.3333333333335, 2333.3333333333335, 2420.0, 2640.0, 2293.3333333333335, 2246.666666666667, 2480.0, 2286.666666666667, 2460.0, 2713.3333333333335, 2466.666666666667, 3506.666666666667, 2853.3333333333335, 2873.3333333333335, 2360.0, 3880.0, 11093.333333333334, 4580.0, 2480.0, 2446.666666666667, 3286.666666666667, 4786.666666666667, 4926.666666666667, 5366.666666666667, 4906.666666666667, 5260.0, 4906.666666666667, 3193.3333333333335, 2646.666666666667, 2473.3333333333335, 2293.3333333333335, 2820.0, 2473.3333333333335, 2706.666666666667, 2526.666666666667, 2466.666666666667, 2900.0, 3940.0, 3973.3333333333335, 4166.666666666667, 2506.666666666667, 2686.666666666667, 2773.3333333333335, 2553.3333333333335, 2446.666666666667, 3133.3333333333335, 2626.666666666667, 2540.0, 2580.0, 2373.3333333333335, 2113.3333333333335, 2053.3333333333335, 2580.0, 2133.3333333333335, 2553.3333333333335, 11513.333333333334, 9366.666666666668, 8800.0, 5600.0, 2366.666666666667, 2513.3333333333335, 2480.0, 2446.666666666667, 2266.666666666667, 2733.3333333333335, 2406.666666666667, 2166.666666666667, 2453.3333333333335, 1873.3333333333335, 2540.0, 2553.3333333333335, 3106.666666666667, 3180.0, 3106.666666666667, 3220.0, 3453.3333333333335, 3546.666666666667, 3073.3333333333335, 2986.666666666667, 3113.3333333333335, 2966.666666666667, 2500.0, 2373.3333333333335, 3306.666666666667, 2540.0, 2806.666666666667, 2413.3333333333335, 2446.666666666667, 2473.3333333333335, 2253.3333333333335, 2126.666666666667, 2620.0, 2086.666666666667, 2153.3333333333335, 2686.666666666667, 2753.3333333333335, 1973.3333333333335, 2200.0, 2326.666666666667, 2386.666666666667, 2133.3333333333335, 2573.3333333333335, 3546.666666666667, 2840.0, 2780.0, 2746.666666666667, 2926.666666666667, 2353.3333333333335, 2846.666666666667, 2500.0, 2626.666666666667, 2493.3333333333335, 2453.3333333333335, 3146.666666666667, 2326.666666666667, 3046.666666666667, 3026.666666666667, 2533.3333333333335, 2100.0, 2513.3333333333335, 3006.666666666667, 2266.666666666667, 2406.666666666667, 1980.0, 2613.3333333333335, 2413.3333333333335, 2393.3333333333335, 2286.666666666667, 2160.0, 2453.3333333333335, 2473.3333333333335, 2640.0, 2153.3333333333335, 2480.0, 2153.3333333333335, 2393.3333333333335, 2313.3333333333335, 2213.3333333333335, 2220.0, 2480.0, 2720.0, 2553.3333333333335, 2506.666666666667, 5120.0, 2446.666666666667, 2346.666666666667, 2526.666666666667, 2773.3333333333335, 2433.3333333333335, 2280.0, 2966.666666666667, 2613.3333333333335, 2806.666666666667, 2893.3333333333335, 2600.0, 2486.666666666667, 3253.3333333333335, 2606.666666666667, 2213.3333333333335, 2566.666666666667, 2466.666666666667, 2660.0, 2740.0, 2480.0, 2100.0, 2706.666666666667, 2766.666666666667, 2600.0, 2346.666666666667, 2860.0, 2400.0, 2726.666666666667, 2933.3333333333335, 2293.3333333333335, 2553.3333333333335, 2426.666666666667, 2320.0, 2380.0, 2620.0, 2726.666666666667, 2553.3333333333335, 2740.0, 2513.3333333333335, 2346.666666666667, 2220.0, 2160.0, 2213.3333333333335, 2480.0, 2346.666666666667, 2426.666666666667, 2553.3333333333335, 2720.0, 2346.666666666667, 2966.666666666667, 2826.666666666667, 2820.0, 2426.666666666667, 2293.3333333333335, 2073.3333333333335, 2566.666666666667, 2813.3333333333335, 2353.3333333333335, 2520.0, 2146.666666666667, 2580.0, 2446.666666666667, 2246.666666666667, 2486.666666666667, 2813.3333333333335, 2400.0, 2626.666666666667, 2186.666666666667, 2626.666666666667, 2560.0, 2693.3333333333335, 3340.0, 2440.0, 2480.0, 2073.3333333333335, 2353.3333333333335, 2406.666666666667, 2546.666666666667, 2806.666666666667, 2840.0, 2193.3333333333335, 2666.666666666667, 2786.666666666667, 2273.3333333333335, 2480.0, 2220.0, 2766.666666666667, 2620.0, 3180.0, 2593.3333333333335, 2673.3333333333335, 2560.0, 2526.666666666667, 2553.3333333333335, 2760.0, 3026.666666666667, 2986.666666666667, 2846.666666666667, 2726.666666666667, 2133.3333333333335, 2360.0, 3053.3333333333335, 2646.666666666667, 2506.666666666667, 2833.3333333333335, 2446.666666666667, 2580.0, 2160.0, 2786.666666666667, 2360.0, 2906.666666666667, 3193.3333333333335, 2326.666666666667, 2766.666666666667, 2273.3333333333335, 3040.0, 2586.666666666667, 3146.666666666667, 3733.3333333333335, 5146.666666666667, 4320.0, 2586.666666666667, 2653.3333333333335, 5440.0, 3953.3333333333335, 2566.666666666667, 2480.0, 2640.0, 2700.0, 2333.3333333333335, 2066.666666666667, 2586.666666666667, 2566.666666666667, 2500.0, 2373.3333333333335, 2680.0, 2240.0, 2880.0, 2173.3333333333335, 2480.0, 2620.0, 2086.666666666667, 2560.0, 2186.666666666667, 2526.666666666667, 1966.6666666666667, 2200.0, 2633.3333333333335, 2280.0, 2253.3333333333335, 2853.3333333333335, 2533.3333333333335, 2146.666666666667, 2366.666666666667, 1980.0, 2106.666666666667, 2460.0, 2060.0, 2566.666666666667, 2020.0, 2693.3333333333335, 2566.666666666667, 2846.666666666667, 2366.666666666667, 2813.3333333333335, 2740.0, 2433.3333333333335, 2860.0, 3453.3333333333335, 2326.666666666667, 2100.0, 2560.0, 2206.666666666667, 2240.0, 2380.0, 2206.666666666667, 2513.3333333333335, 2600.0, 2673.3333333333335, 2980.0, 2480.0, 2280.0, 2846.666666666667, 2746.666666666667, 2386.666666666667, 2466.666666666667, 2433.3333333333335, 2880.0, 3213.3333333333335, 2406.666666666667, 2986.666666666667, 2913.3333333333335, 2313.3333333333335, 2020.0, 2060.0, 2326.666666666667, 2173.3333333333335, 2540.0, 2326.666666666667, 2100.0, 2353.3333333333335, 2360.0, 1920.0, 2720.0, 2740.0, 2880.0, 2880.0, 5586.666666666667, 3140.0, 2220.0, 2346.666666666667, 2313.3333333333335, 2606.666666666667, 2686.666666666667, 2333.3333333333335, 2333.3333333333335, 2146.666666666667, 2573.3333333333335, 2400.0, 2453.3333333333335, 2400.0, 2026.6666666666667, 2740.0], [180.0, 266.6666666666667, 233.33333333333334, 133.33333333333334, 253.33333333333334, 213.33333333333334, 240.0, 173.33333333333334, 240.0, 140.0, 146.66666666666669, 266.6666666666667, 233.33333333333334, 193.33333333333334, 233.33333333333334, 220.0, 173.33333333333334, 173.33333333333334, 240.0, 220.0, 173.33333333333334, 193.33333333333334, 220.0, 253.33333333333334, 253.33333333333334, 140.0, 193.33333333333334, 186.66666666666669, 193.33333333333334, 133.33333333333334, 213.33333333333334, 180.0, 293.33333333333337, 173.33333333333334, 253.33333333333334, 240.0, 240.0, 273.33333333333337, 193.33333333333334, 226.66666666666669, 213.33333333333334, 133.33333333333334, 206.66666666666669, 253.33333333333334, 253.33333333333334, 206.66666666666669, 200.0, 200.0, 200.0, 193.33333333333334, 253.33333333333334, 320.0, 166.66666666666669, 246.66666666666669, 253.33333333333334, 166.66666666666669, 253.33333333333334, 186.66666666666669, 206.66666666666669, 206.66666666666669, 233.33333333333334, 213.33333333333334, 186.66666666666669, 273.33333333333337, 286.6666666666667, 253.33333333333334, 120.0, 160.0, 166.66666666666669, 240.0, 180.0, 233.33333333333334, 220.0, 286.6666666666667, 166.66666666666669, 186.66666666666669, 220.0, 253.33333333333334, 226.66666666666669, 200.0, 293.33333333333337, 286.6666666666667, 273.33333333333337, 373.33333333333337, 353.33333333333337, 580.0, 713.3333333333334, 486.6666666666667, 813.3333333333334, 853.3333333333334, 860.0, 826.6666666666667, 800.0, 1386.6666666666667, 900.0, 1053.3333333333335, 986.6666666666667, 940.0, 953.3333333333334, 1186.6666666666667, 926.6666666666667, 846.6666666666667, 966.6666666666667, 840.0, 1073.3333333333335, 853.3333333333334, 1013.3333333333334, 880.0, 926.6666666666667, 900.0, 913.3333333333334, 960.0, 873.3333333333334, 960.0, 1053.3333333333335, 1146.6666666666667, 886.6666666666667, 746.6666666666667, 1026.6666666666667, 940.0, 800.0, 1106.6666666666667, 980.0, 1053.3333333333335, 986.6666666666667, 880.0, 1093.3333333333335, 980.0, 753.3333333333334, 873.3333333333334, 813.3333333333334, 900.0, 993.3333333333334, 986.6666666666667, 866.6666666666667, 1053.3333333333335, 846.6666666666667, 853.3333333333334, 986.6666666666667, 893.3333333333334, 966.6666666666667, 1020.0, 900.0, 1080.0, 1086.6666666666667, 1093.3333333333335, 1006.6666666666667, 920.0, 1000.0, 1053.3333333333335, 1173.3333333333335, 1066.6666666666667, 780.0, 760.0, 713.3333333333334, 893.3333333333334, 760.0, 913.3333333333334, 780.0, 946.6666666666667, 973.3333333333334, 933.3333333333334, 933.3333333333334, 993.3333333333334, 1113.3333333333335, 953.3333333333334, 1033.3333333333335, 800.0, 906.6666666666667, 913.3333333333334, 946.6666666666667, 853.3333333333334, 1040.0, 1040.0, 886.6666666666667, 946.6666666666667, 860.0, 820.0, 1226.6666666666667, 946.6666666666667, 960.0, 1126.6666666666667, 1113.3333333333335, 1006.6666666666667, 813.3333333333334, 1040.0, 1020.0, 920.0, 860.0, 1066.6666666666667, 1120.0, 1066.6666666666667, 980.0, 866.6666666666667, 1006.6666666666667, 820.0, 946.6666666666667, 2400.0, 1093.3333333333335, 1140.0, 1026.6666666666667, 1140.0, 973.3333333333334, 1120.0, 1026.6666666666667, 953.3333333333334, 980.0, 940.0, 1086.6666666666667, 813.3333333333334, 1146.6666666666667, 1506.6666666666667, 1186.6666666666667, 1206.6666666666667, 1273.3333333333335, 993.3333333333334, 1006.6666666666667, 1140.0, 973.3333333333334, 1093.3333333333335, 953.3333333333334, 1060.0, 1013.3333333333334, 1093.3333333333335, 1186.6666666666667, 1066.6666666666667, 866.6666666666667, 886.6666666666667, 1093.3333333333335, 893.3333333333334, 866.6666666666667, 853.3333333333334, 1040.0, 1040.0, 826.6666666666667, 1093.3333333333335, 973.3333333333334, 926.6666666666667, 1046.6666666666667, 1773.3333333333335, 840.0, 853.3333333333334, 1186.6666666666667, 846.6666666666667, 880.0, 813.3333333333334, 1073.3333333333335, 886.6666666666667, 966.6666666666667, 920.0, 933.3333333333334, 1013.3333333333334, 900.0, 1026.6666666666667, 1266.6666666666667, 953.3333333333334, 906.6666666666667, 1026.6666666666667, 946.6666666666667, 946.6666666666667, 1140.0, 960.0, 1400.0, 1020.0, 1133.3333333333335, 1186.6666666666667, 1106.6666666666667, 800.0, 866.6666666666667, 1073.3333333333335, 1593.3333333333335, 1006.6666666666667, 1173.3333333333335, 960.0, 813.3333333333334, 1146.6666666666667, 933.3333333333334, 933.3333333333334, 920.0, 1060.0, 986.6666666666667, 1100.0, 1120.0, 806.6666666666667, 1073.3333333333335, 1040.0, 813.3333333333334, 953.3333333333334, 1433.3333333333335, 926.6666666666667, 1140.0, 1020.0, 973.3333333333334, 1033.3333333333335, 886.6666666666667, 866.6666666666667, 920.0, 980.0, 1426.6666666666667, 960.0, 913.3333333333334, 926.6666666666667, 966.6666666666667, 1040.0, 1086.6666666666667, 1033.3333333333335, 1120.0, 1193.3333333333335, 1040.0, 966.6666666666667, 1206.6666666666667, 966.6666666666667, 993.3333333333334, 1166.6666666666667, 933.3333333333334, 846.6666666666667, 900.0, 1013.3333333333334, 906.6666666666667, 893.3333333333334, 1073.3333333333335, 880.0, 926.6666666666667, 953.3333333333334, 880.0, 1040.0, 773.3333333333334, 900.0, 906.6666666666667, 1000.0, 1153.3333333333335, 1033.3333333333335, 993.3333333333334, 840.0, 1020.0, 980.0, 953.3333333333334, 786.6666666666667, 1033.3333333333335, 853.3333333333334, 1000.0, 1340.0, 1213.3333333333335, 1040.0, 873.3333333333334, 973.3333333333334, 993.3333333333334, 1040.0, 940.0, 986.6666666666667, 1006.6666666666667, 866.6666666666667, 1006.6666666666667, 1046.6666666666667, 906.6666666666667, 900.0, 946.6666666666667, 1040.0, 873.3333333333334, 913.3333333333334, 1053.3333333333335, 1040.0, 893.3333333333334, 966.6666666666667, 1246.6666666666667, 1126.6666666666667, 1046.6666666666667, 986.6666666666667, 946.6666666666667, 1053.3333333333335, 1126.6666666666667, 953.3333333333334, 973.3333333333334, 946.6666666666667, 993.3333333333334, 826.6666666666667, 986.6666666666667, 1200.0, 920.0, 1053.3333333333335, 1000.0, 933.3333333333334, 906.6666666666667, 1193.3333333333335, 793.3333333333334, 1033.3333333333335, 980.0, 886.6666666666667, 1273.3333333333335, 1093.3333333333335, 766.6666666666667, 826.6666666666667, 880.0, 833.3333333333334, 920.0, 1313.3333333333335, 1046.6666666666667, 1026.6666666666667, 1033.3333333333335, 1093.3333333333335, 926.6666666666667, 1026.6666666666667, 866.6666666666667, 886.6666666666667, 1053.3333333333335, 993.3333333333334, 1080.0, 1033.3333333333335, 946.6666666666667, 993.3333333333334, 1240.0, 1253.3333333333335, 1033.3333333333335, 1166.6666666666667, 1060.0, 1133.3333333333335, 1106.6666666666667, 1160.0, 1073.3333333333335, 866.6666666666667, 1086.6666666666667, 1046.6666666666667, 1080.0, 1033.3333333333335, 1166.6666666666667, 1066.6666666666667, 980.0, 1066.6666666666667, 1053.3333333333335, 1140.0, 893.3333333333334, 973.3333333333334, 993.3333333333334, 1113.3333333333335, 1093.3333333333335, 1080.0, 1060.0, 933.3333333333334, 1080.0, 973.3333333333334, 1013.3333333333334, 1020.0, 933.3333333333334, 1120.0, 926.6666666666667, 953.3333333333334, 1080.0, 1713.3333333333335, 1100.0, 973.3333333333334, 940.0, 840.0, 1126.6666666666667, 1000.0, 906.6666666666667, 1053.3333333333335, 926.6666666666667, 853.3333333333334, 893.3333333333334, 953.3333333333334, 980.0, 1426.6666666666667, 986.6666666666667, 1040.0, 900.0, 960.0, 1000.0, 1040.0, 900.0, 986.6666666666667, 973.3333333333334, 860.0, 1020.0, 1000.0, 840.0, 1000.0, 913.3333333333334, 973.3333333333334, 1033.3333333333335, 800.0, 960.0, 1113.3333333333335, 933.3333333333334, 913.3333333333334, 1053.3333333333335, 953.3333333333334, 986.6666666666667, 1046.6666666666667, 1133.3333333333335, 1046.6666666666667, 1033.3333333333335, 1813.3333333333335, 853.3333333333334, 973.3333333333334, 1213.3333333333335, 1093.3333333333335, 820.0, 806.6666666666667, 1026.6666666666667, 966.6666666666667, 733.3333333333334, 980.0, 846.6666666666667, 946.6666666666667, 1113.3333333333335, 766.6666666666667, 1020.0, 960.0, 940.0, 1006.6666666666667, 946.6666666666667, 1306.6666666666667, 800.0, 866.6666666666667, 953.3333333333334, 933.3333333333334, 1006.6666666666667, 1113.3333333333335, 866.6666666666667, 853.3333333333334, 793.3333333333334, 826.6666666666667, 980.0, 866.6666666666667, 833.3333333333334, 1100.0, 1133.3333333333335, 1013.3333333333334, 1200.0, 880.0, 1073.3333333333335, 920.0, 966.6666666666667, 1040.0, 953.3333333333334, 973.3333333333334, 780.0, 786.6666666666667, 933.3333333333334, 940.0, 960.0, 860.0, 866.6666666666667, 966.6666666666667, 780.0, 866.6666666666667, 913.3333333333334, 980.0, 953.3333333333334, 1093.3333333333335, 1080.0, 1313.3333333333335, 873.3333333333334, 1013.3333333333334, 800.0, 900.0, 1020.0, 1126.6666666666667, 833.3333333333334, 1160.0, 1073.3333333333335, 1120.0, 1020.0, 1040.0, 1000.0, 1113.3333333333335, 1000.0, 980.0, 800.0, 1073.3333333333335, 1140.0, 966.6666666666667, 1026.6666666666667, 1000.0, 786.6666666666667, 1006.6666666666667, 1166.6666666666667, 933.3333333333334, 973.3333333333334, 1053.3333333333335, 973.3333333333334, 860.0, 1373.3333333333335, 1073.3333333333335, 946.6666666666667, 966.6666666666667, 973.3333333333334, 1226.6666666666667, 820.0, 900.0, 906.6666666666667, 820.0, 953.3333333333334, 1066.6666666666667, 826.6666666666667, 1200.0, 920.0, 1053.3333333333335, 1166.6666666666667, 1020.0, 1020.0, 946.6666666666667, 993.3333333333334, 993.3333333333334, 1013.3333333333334, 933.3333333333334, 960.0, 813.3333333333334, 1006.6666666666667, 946.6666666666667, 926.6666666666667, 1446.6666666666667, 1053.3333333333335, 926.6666666666667, 960.0, 1106.6666666666667, 820.0, 1093.3333333333335, 1013.3333333333334, 873.3333333333334, 986.6666666666667, 1086.6666666666667, 1040.0, 1153.3333333333335, 980.0, 740.0, 973.3333333333334, 980.0, 1473.3333333333335, 1093.3333333333335, 1033.3333333333335, 1093.3333333333335, 920.0, 780.0, 1153.3333333333335, 1380.0, 840.0, 1100.0, 966.6666666666667, 973.3333333333334, 1033.3333333333335, 800.0, 853.3333333333334, 1066.6666666666667, 940.0, 953.3333333333334, 926.6666666666667, 946.6666666666667, 1073.3333333333335, 986.6666666666667, 900.0, 860.0, 920.0, 960.0, 1060.0, 980.0, 880.0, 1026.6666666666667, 853.3333333333334, 906.6666666666667, 1166.6666666666667, 1100.0, 946.6666666666667, 1013.3333333333334, 1000.0, 1033.3333333333335, 933.3333333333334, 1093.3333333333335, 1126.6666666666667, 873.3333333333334, 1006.6666666666667, 940.0, 1060.0, 1106.6666666666667, 1086.6666666666667, 1020.0, 1026.6666666666667, 1113.3333333333335, 920.0, 866.6666666666667, 1093.3333333333335, 1066.6666666666667, 1000.0, 1146.6666666666667, 900.0, 873.3333333333334, 1093.3333333333335, 1073.3333333333335, 1073.3333333333335, 1060.0, 1073.3333333333335, 1606.6666666666667, 1333.3333333333335, 813.3333333333334, 1073.3333333333335, 1046.6666666666667, 
